vi "VerifyArrayOfClustersWithStrings.vi"(11 "Input Array":T1(array[cluster])) -> (3 "Arrays Are Equal?":bool)   [LabVIEW 2010]
panel:
  in  "Expected Array":T1(array[cluster])=[{"New String"="Foo - TestStand Rules", "Has All Array 1 Strings Concatenated"="AAA_BBB_ - TestStand Rules", "Array"=["AAA_", "BBB_", " - TestStand Rules"], "Array 2"=["a", "b", "c"], "String 2"="Not A Default Value"}, {"New String"="Go Cowboys!", "Has All Array 1 Strings Concatenated"="How_About_Them_ Cowboys!", "Array"=["How_", "About_", "Them_", " Cowboys!"], "Array 2"=["Foo", "Bar"], "String 2"="FooBar"}, {"New String"="Los Vaqueros!", "Has All Array 1 Strings Concatenated"="Que_Tal_Esos_ Vaqueros!", "Array"=["Que_", "Tal_", "Esos_", " Vaqueros!"], "Array 2"=["Vamos", " Vaqueros!"], "String 2"="Esta en blanco"}]
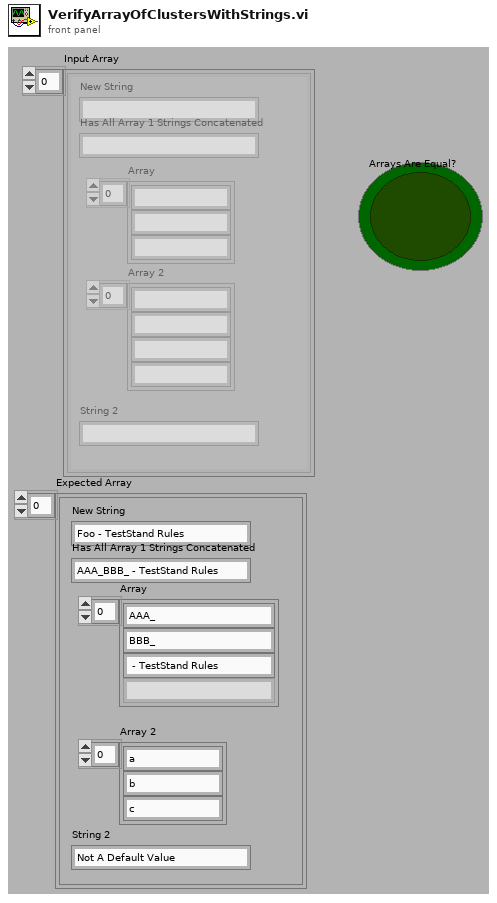
[diagram p1: front panel]
types:
  T1 = cluster{"New String":string, "Has All Array 1 Strings Concatenated":string, "Array":string[], "Array 2":string[], "String 2":string}[]
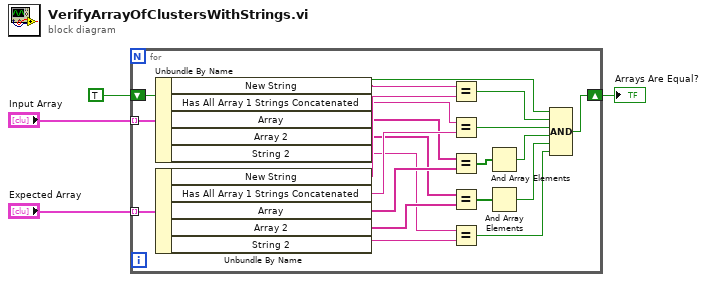
[diagram p0: block diagram]
diagram:
  n1 = for {
    tunnel: "Input Array" -> [w25] mode=indexing
    tunnel: "Expected Array" -> [w24] mode=indexing
    shift-right: [w11] -> w1
    shift-left: TRUE -> [w10]
    n2 = Unbundle By Name(w25) -> ("New String"=w23:string, "Has All Array 1 Strings Concatenated"=w21:string, "Array"=w19:string[], "Array 2"=w17:string[], "String 2"=w14:string)
    n3 = Unbundle By Name(w24) -> ("New String"=w22:string, "Has All Array 1 Strings Concatenated"=w20:string, "Array"=w18:string[], "Array 2"=w16:string[], "String 2"=w15:string)
    n4 = Equal?(x=w23, y=w22) -> (x = y?=w9:bool)
    n5 = Equal?(x=w21, y=w20) -> (x = y?=w8:bool)
    n6 = Equal?(x=w19, y=w18) -> (x = y?=w13:bool[])
    n7 = Equal?(x=w17, y=w16) -> (x = y?=w12:bool[])
    n8 = Equal?(x=w14, y=w15) -> (x = y?=w5:bool)
    n9 = And Array Elements(Boolean array=w13) -> (logical AND=w7:bool)
    n10 = And Array Elements(Boolean array=w12) -> (logical AND=w6:bool)
    n11 = Compound Arithmetic op=AND(w10, w9, w8, w7, w6, w5) -> (w11:bool)
  }
  "Arrays Are Equal?" <- w1
